vi "DisconnectCamera.vi"(8 "error in (no error)":errorcluster, 11 "CameraTestingBL in":refnum<class "CameraTesting.lvclass">) -> (0 "error out":errorcluster, 3 "CameraTestingBL out":refnum<class "CameraTesting.lvclass">)   [LabVIEW 2020, in "CameraTesting.lvlib" / "CameraTesting.lvclass"]
doc: "disconnect to camera"
uses:
  CameraTesting.lvclass
  CameraTesting.lvclass/CameraTesting.ctl
  <vilib>/ActorFramework/Message Enqueuer/Message Enqueuer.lvclass/Message Enqueuer.ctl
  <vilib>/ActorFramework/Message Enqueuer/Enqueue.vi
  ICameraTestingUI/ICameraTestingUI Messages/DisconnectCameraRslt Msg/DisconnectCameraRslt Msg.lvclass
  C:/Program Files (x86)/National Instruments/LabVIEW 2020/vi.lib/ActorFramework/Message/Message.lvclass
  <vilib>/ActorFramework/Message Priority Queue/Priority Enqueue.vi
  Camera/ICamera/ICamera/ICamera.lvclass
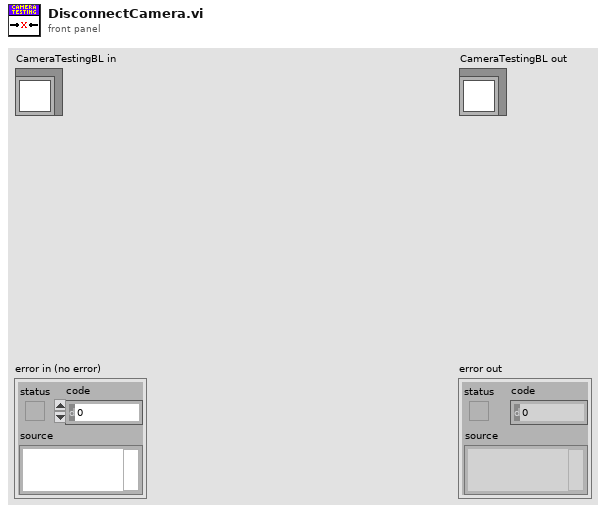
[diagram p1: front panel]
types:
  T1 = typedef "ICameraTesting.lvlib/ICameraTesting.lvclass/StatusUpdated.ctl" = refnum<user-event>
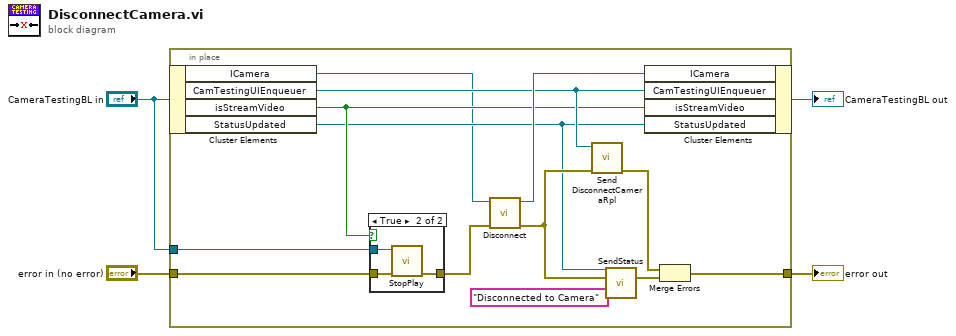
[diagram p0: block diagram]
diagram:
  n1 = in-place {
    in-place-border: [w10] -> w4
    in-place-border: "error in (no error)" -> [w13]
    in-place-border: "CameraTestingBL in" -> [w8]
    n2 = in-place-cluster #1("CameraTestingBL in") -> ("ICamera"=w6:refnum<class "ICamera.lvclass">, "CamTestingUIEnqueuer"=w16:refnum<class "Message Enqueuer.lvclass">, "isStreamVideo"=w14:bool, "StatusUpdated"=w11:T1)
    n3 = case shown="True" w14 {
      tunnel: w13 -> [w18 w20]
      tunnel: [w18 w19] -> w7
      tunnel: w8 -> [_ w21]
      frame False {
      }
      frame True {
        n4 = call-dynamic "StopPlay.vi"("error in (no error)"=w20, "CameraTestingBL in"=w21) -> ("error out"=w19:errorcluster)  [unwired: 8 in, 1 out]
      }
    }
    n5 = call-dynamic "Disconnect.vi"("error in (no error)"=w7, "ICamera in"=w6) -> ("error out"=w12:errorcluster, "ICamera out"=w17:refnum<class "ICamera.lvclass">)  [unwired: 8 in]
    n6 = call "Send DisconnectCameraRpl.vi"("error in (no error)"=w12, "Message Enqueuer"=w16) -> ("error out"=w15:errorcluster)  [unwired: 8 in, 1 out]
    n7 = call "SendStatus.vi"("StatusUsrEvn"=w11, "error in"=w12, "Text"="Disconnected to Camera") -> ("error out"=w9:errorcluster)  [unwired: 24 in]
    n8 = in-place-cluster #1("ICamera"=w17, "CamTestingUIEnqueuer"=w16, "isStreamVideo"=w14, "StatusUpdated"=w11) -> (→"CameraTestingBL out":refnum<class "CameraTesting.lvclass">)
    n9 = Merge Errors(w15, w9) -> (w10:errorcluster)
  }
  "error out" <- w4
